vi "test.vi"() -> ()   [LabVIEW 2022 SP3, in "SingleStepTestV3.lvlib" / "SingleStepTestV3.lvclass"]
uses:
  SingleStepTestV3.lvclass
panel:
  in  "单步调试":T9={"注射泵"=enum."注入", "阀口选择"=enum."V1", "灯"=enum."未选择", "ADC值"=enum."未选择", "数值"=4000, "项目输入"=0, "控温"={"氨氮控温"=FALSE, "消解"=FALSE, "恒温"=FALSE, "降温"=FALSE}, "外设选择"={"蠕动泵"=FALSE, "电磁阀1"=FALSE, "电磁阀2"=FALSE, "慢速"=FALSE}, "外设选择2"={"V9-1"=FALSE, "V9-2"=FALSE, "顺时针"=FALSE, "逆时针"=FALSE}, "反滴定"=FALSE, "试剂检测"=FALSE} {"项目输入" items=["总磷"=1, "总氮"=2, "氨氮"=3, "磷酸盐"=4, "硝氮"=5, "亚硝氮"=6, "硅酸盐"=7, "硫化物"=8, "CODcr"=22, "氟化物"=50]}
  in  "仪器版本":T10=enum."V4版"
  out "数组":u16[](array[numeric]) format="%04x"
  in  "布尔":bool
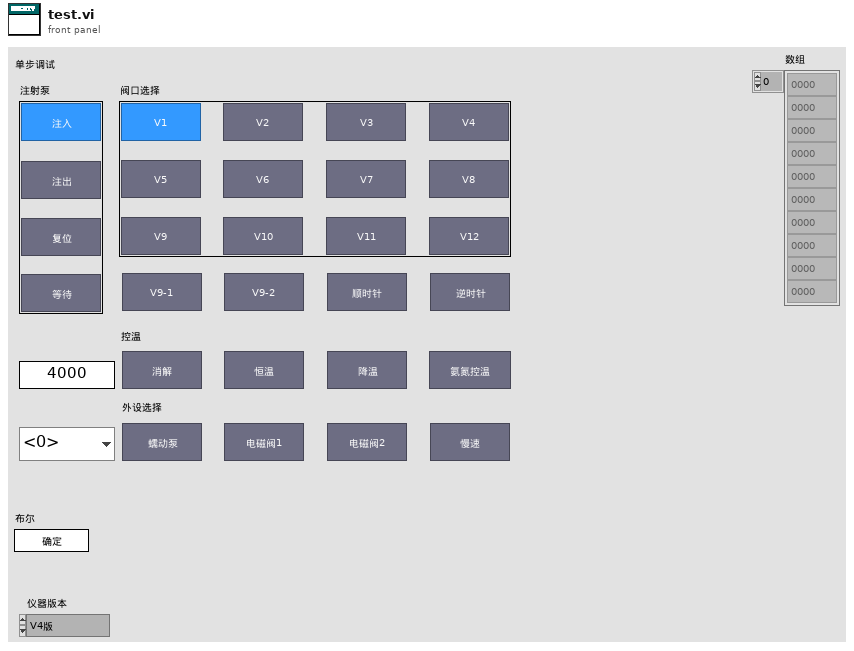
[diagram p1: front panel]
types:
  T1 = typedef "SingleStepTestV3.lvlib/SingleStepTestV3.lvclass/注射泵操作.ctl" = enum32{"复位", "注入", "注出", "等待"}
  T2 = typedef "SingleStepTestV3.lvlib/SingleStepTestV3.lvclass/阀口操作.ctl" = enum32{"未选择", "V1", "V2", "V3", "V4", "V5", "V6", "V7", "V8", "V9", "V10", "V11", "V12"}
  T3 = typedef "SingleStepTestV3.lvlib/SingleStepTestV3.lvclass/灯选择.ctl" = enum32{"未选择", "365", "520", "660", "氙灯/紫灯"}
  T4 = typedef "SingleStepTestV3.lvlib/SingleStepTestV3.lvclass/ADC选择.ctl" = enum32{"未选择", "ADC365", "ADC520", "ADC660", "光谱仪"}
  T5 = typedef "SingleStepTestV3.lvlib/SingleStepTestV3.lvclass/控温操作.ctl" = cluster{"氨氮控温":bool, "消解":bool, "恒温":bool, "降温":bool}
  T6 = typedef "SingleStepTestV3.lvlib/SingleStepTestV3.lvclass/外设选择.ctl" = cluster{"蠕动泵":bool, "电磁阀1":bool, "电磁阀2":bool, "慢速":bool}
  T7 = typedef "SingleStepTestV3.lvlib/SingleStepTestV3.lvclass/外设选择2.ctl" = cluster{"V9-1":bool, "V9-2":bool, "顺时针":bool, "逆时针":bool}
  T8 = typedef "SingleStepTestV3.lvlib/SingleStepTestV3.lvclass/布尔按钮.ctl" = bool
  T9 = cluster{"注射泵":T1, "阀口选择":T2, "灯":T3, "ADC值":T4, "数值":i16, "项目输入":u16, "控温":T5, "外设选择":T6, "外设选择2":T7, "反滴定":T8, "试剂检测":T8}
  T10 = typedef "SingleStepTestV3.lvlib/SingleStepTestV3.lvclass/仪器版本.ctl" = enum16{"V3.1版", "V4版", "V3版", "V4.2版"}
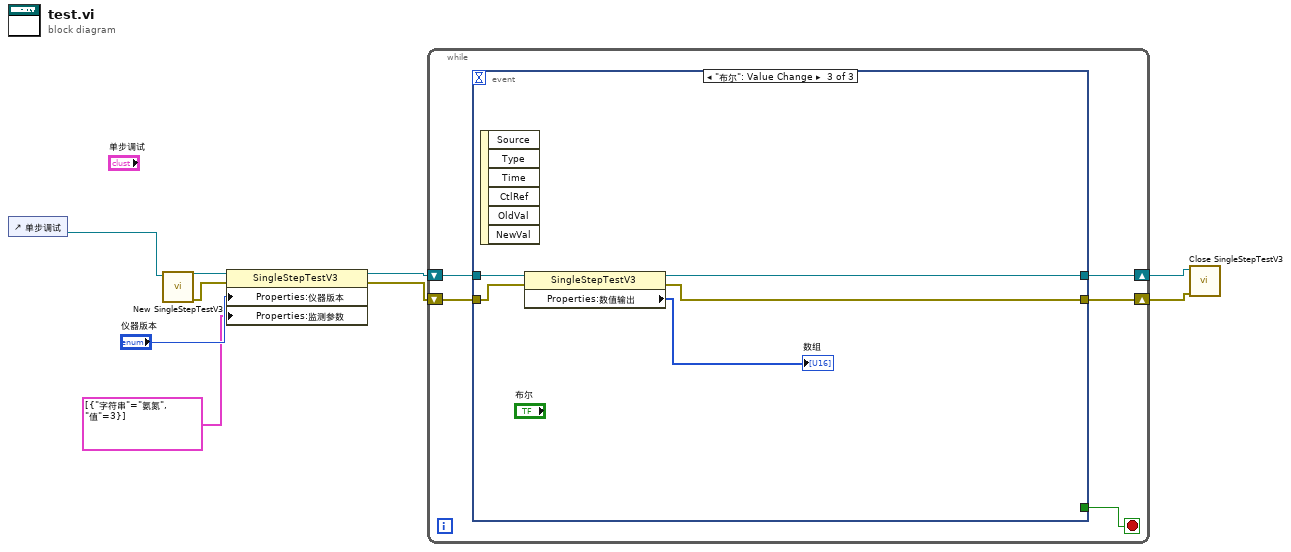
[diagram p0: block diagram]
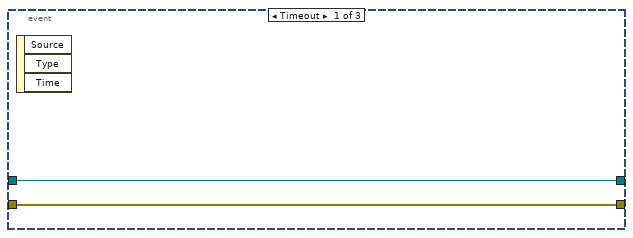
[diagram p2: hidden frame]
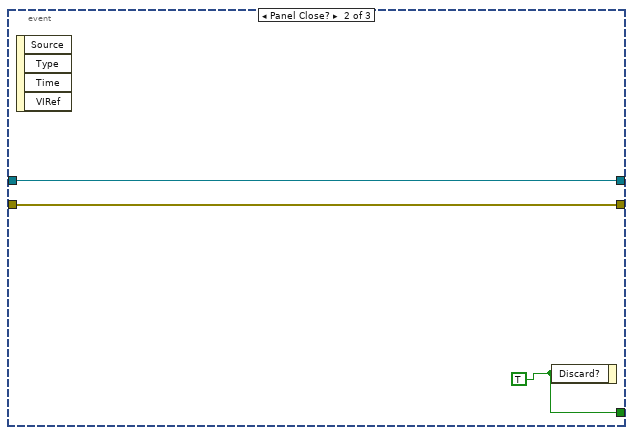
[diagram p3: hidden frame]
diagram:
  n1 = control-ref of="单步调试"() -> (w1:refnum<vi>)
  n2 = call "New SingleStepTestV3.vi"("Reference"=w1) -> ("error out"=w7:errorcluster, "SingleStepTestV3 out"=w2:refnum<class "SingleStepTestV3.lvclass">)  [unwired: 9 in]
  n3 = property class="SingleStepTestV3"(reference=w2, error in=w7, "Properties:仪器版本"="仪器版本", "Properties:监测参数"=cluster{"字符串":string, "值":u16}[] [{"字符串"="氨氮", "值"=3}] ("字符串与值")) -> (reference out=w6:refnum<class "SingleStepTestV3.lvclass">, error out=w5:errorcluster)
  n4 = while {
    shift-right: [w11] -> w9
    shift-left: w6 -> [w14]
    shift-right: [w10] -> w8
    shift-left: w5 -> [w13]
    stop <- w12 stop-if-true
    n5 = event shown="[2] \"布尔\": Value Change" {
      selector: _ -> [_ _ _]
      dyn-events: _ -> [_ _ _]
      timeout: _ -> [_ _ _]
      tunnel: w14 -> [w16 w18 w24]
      tunnel: w13 -> [w15 w17 w20]
      tunnel: [_ w19 _] -> w12
      tunnel: [w16 w18 w23] -> w11
      tunnel: [w15 w17 w22] -> w10
      event Timeout {
        n6 = event-data() -> ()  [unwired: 1 in, 3 out]
      }
      event Panel Close? {
        w19 = TRUE
        n7 = event-data() -> ()  [unwired: 1 in, 4 out]
        n8 = event-data("Discard?"=w19) -> ()  [unwired: 1 in, 1 out]
      }
      event "布尔": Value Change {
        n9 = event-data() -> ()  [unwired: 1 in, 6 out]
        n10 = property class="SingleStepTestV3"(reference=w24, error in=w20) -> (reference out=w23:refnum<class "SingleStepTestV3.lvclass">, error out=w22:errorcluster, "Properties:数值输出"=→"数组":u16[])
      }
    }
  }
  n11 = call "Close SingleStepTestV3.vi"("error in (no error)"=w8, "SingleStepTestV3 in"=w9) -> ()  [unwired: 9 in, 1 out]
